vi "microwaves.vi"(7 "override":bool, 8 "error in (no error)":errorcluster, 10 "frequency (GHz)":dbl=31.95, 11 "VISA IN":refnum<visa-resource-name>) -> (0 "error out":errorcluster, 3 "value out":dbl format="%#_6p")   [LabVIEW 2017]
panel:
  in  "VISA (default)":refnum<visa-resource-name>="mu_wave"
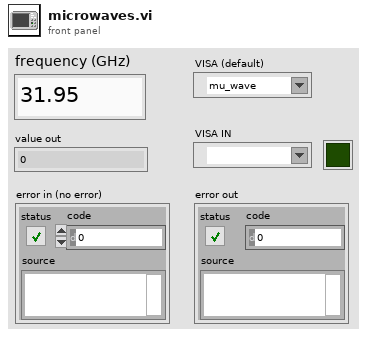
[diagram p1: front panel]
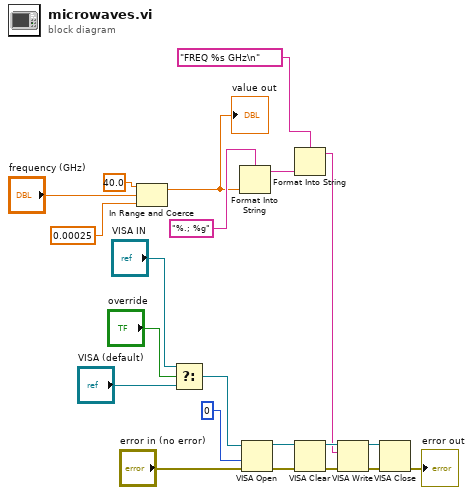
[diagram p0: block diagram]
diagram:
  n1 = In Range and Coerce(upper limit=40.0, x="frequency (GHz)", lower limit=0.00025 ("x")) -> (coerced(x)=w5:dbl)  [unwired: 1 out]
  "value out" <- w5
  n2 = Select(t="VISA IN", s="override", f="VISA (default)") -> (s? t:f=w1:refnum<visa-resource-name>)
  n3 = Format Into String(format string="%.; %g", w5) -> (resulting string=w10:string)  [unwired: 2 in, 1 out]
  n4 = VISA Open(access mode=u32 0, error in (no error)="error in (no error)", VISA resource name=w1) -> (VISA resource name=w20:refnum<visa-resource-name>, error out=w19:errorcluster)  [unwired: 2 in]
  n5 = Format Into String(format string="FREQ %s GHz\n", w10) -> (resulting string=w11:string)  [unwired: 2 in, 1 out]
  n6 = VISA Clear(VISA resource name=w20, error in (no error)=w19) -> (VISA resource name out=w17:refnum<visa-resource-name>, error out=w16:errorcluster)
  n7 = VISA Write(VISA resource name=w17, write buffer=w11, error in (no error)=w16) -> (VISA resource name out=w15:refnum<visa-resource-name>, error out=w14:errorcluster)  [unwired: 1 out]
  n8 = VISA Close(VISA resource name=w15, error in (no error)=w14) -> (error out=→"error out":errorcluster)
